vi "BIAS_Wrapper.vi"() -> ()   [LabVIEW 2012]
uses:
  <userlib>/bias2/subvis/ui/CameraParameters.ctl
  <userlib>/_OpenG.lib/array/array.llb/Search 1D Array (Boolean)__ogtk.vi
panel:
  in  "Labconfig file":path=path "C:/labconfig/ianspielman9339.ini"
  out "zlock port":u32=7339
  out "zlock server":string="atomchip-1.nist.gov"
  out "Current Camera":i32
  in  "Camera Select":i32(c297)
  out "Started":bool=TRUE
  out "VI refs":refnum<vi>[](array[refnum])
  in  "Location of BIAS vi":path=path "C:/Program Files (x86)/National Instruments/LabVIEW 2012/user.lib/BIAS2/BIAS_Client.vi"
  in  "offline":bool
  out "h5 file":path=path "C:/Experiments/rb_chip/connectiontable.h5"
  in  "cancel":bool
  in  "connect":bool
  in  "cameras":i32[](listbox)=[1]
  # "Global configuration options"
  # "Select camera(s) to connect to:"
  # "Loaded config information"
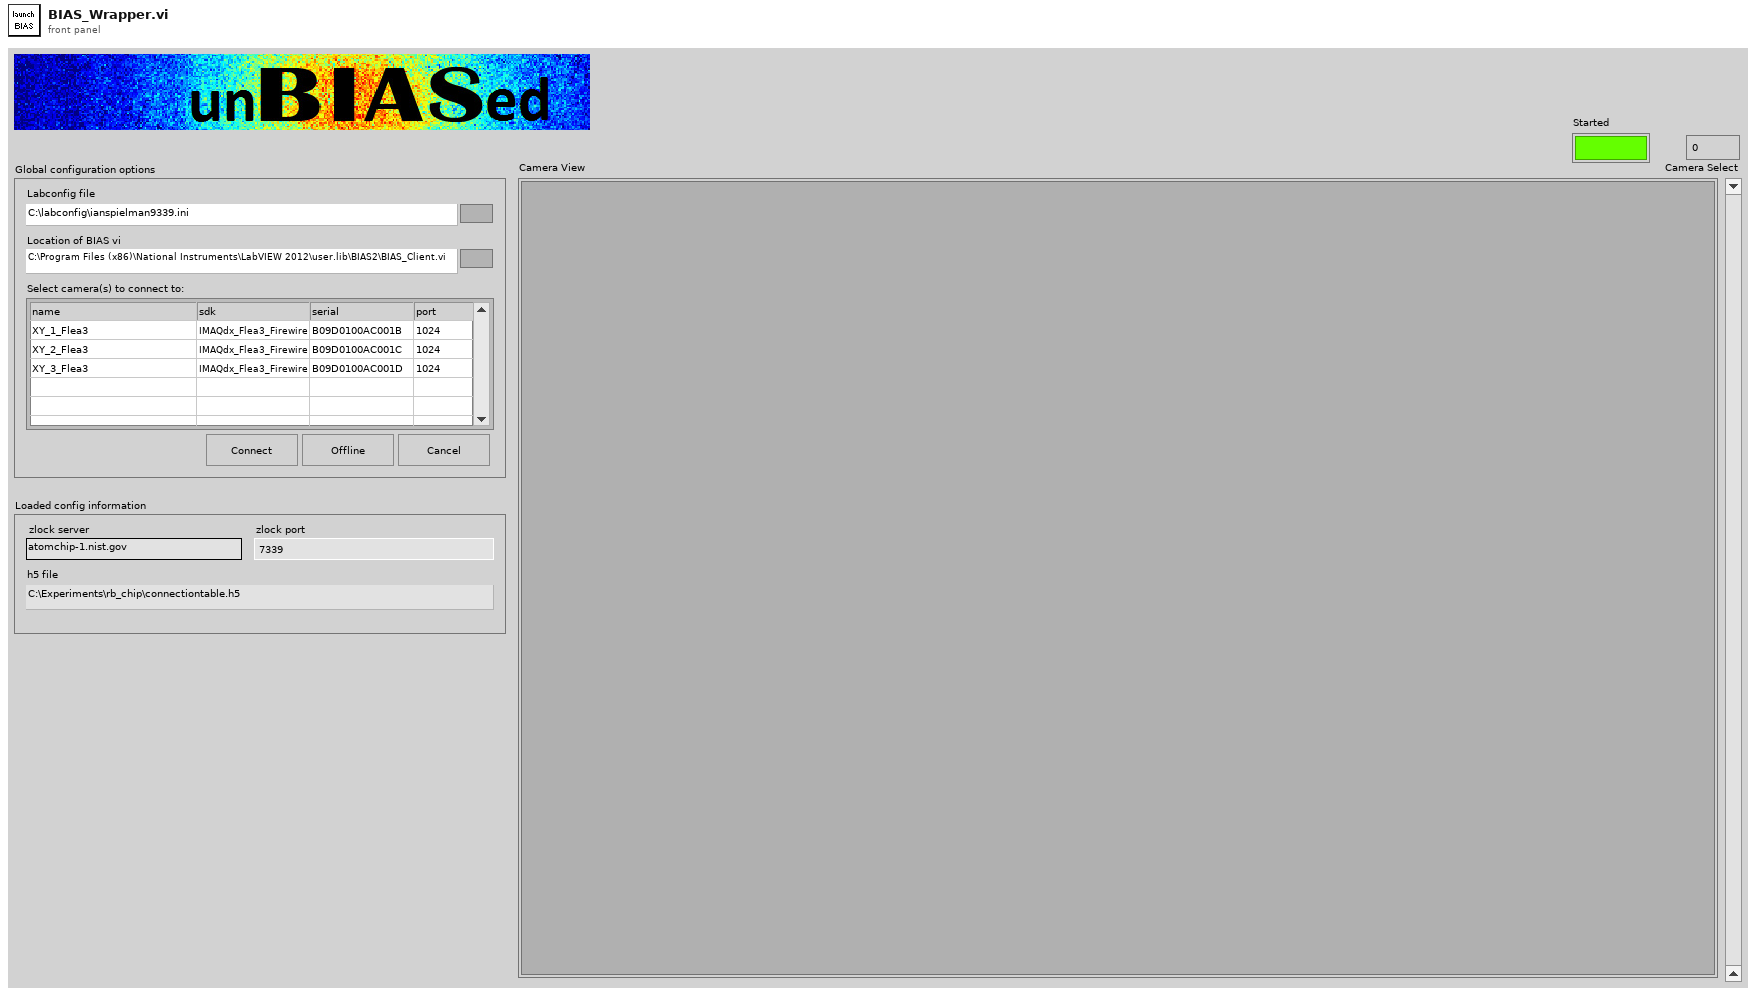
[diagram p1: front panel]
types:
  T1 = typedef "CameraParameters.ctl" = cluster{"name":string, "sdk":string, "serial":u64, "port":u16, "h5":path, "zlock server":string, "zlock port":u32}
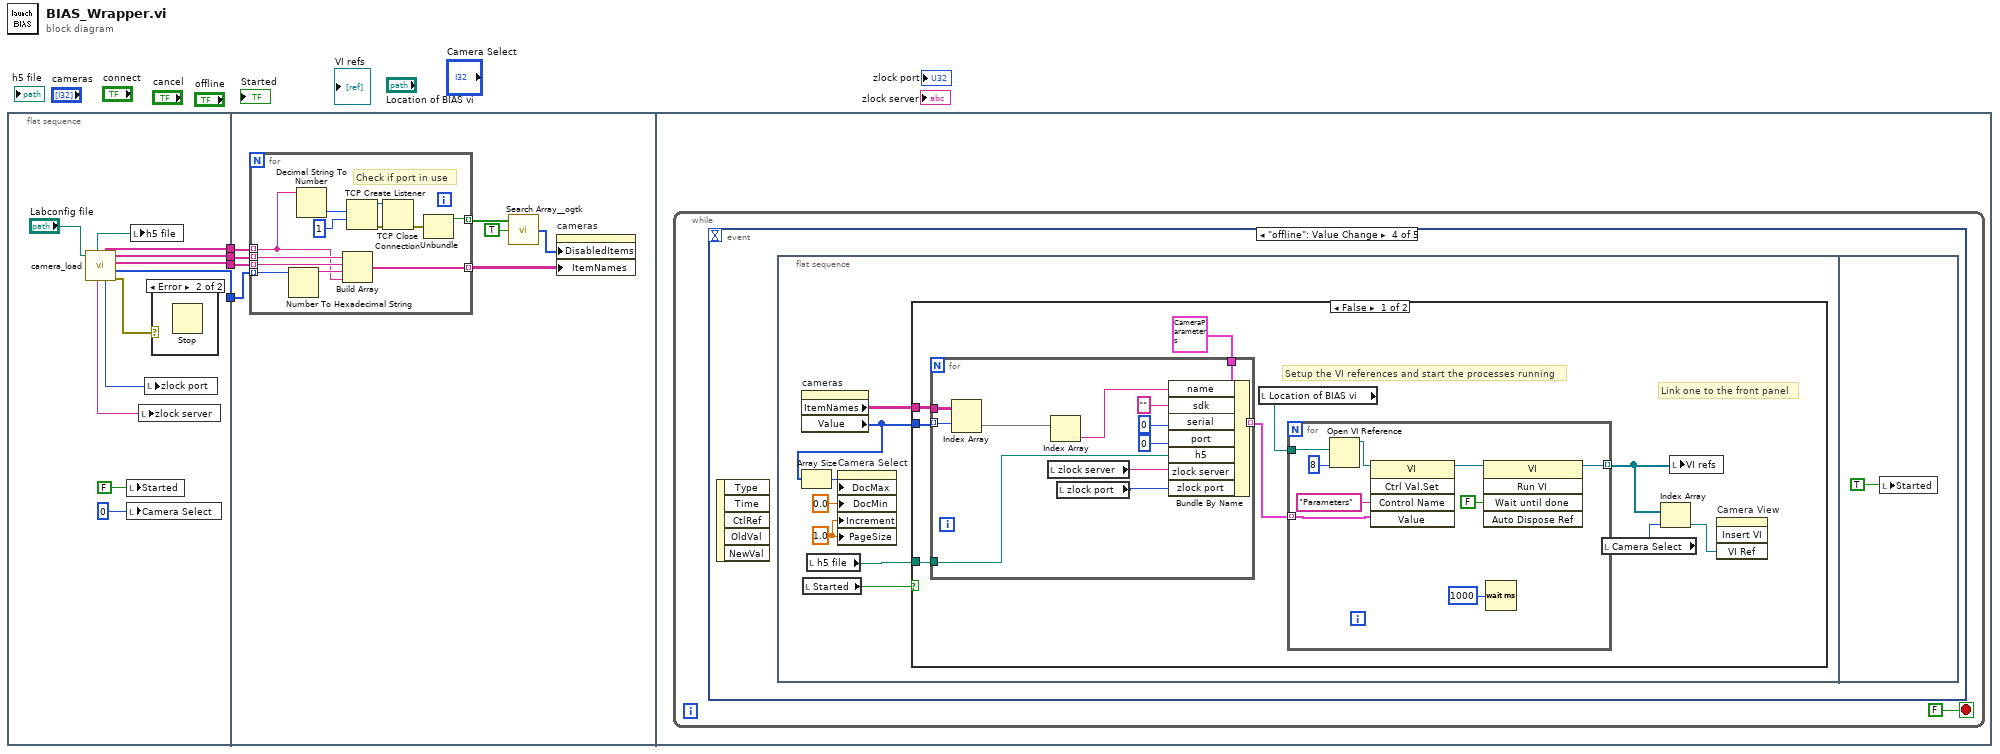
[diagram p0: block diagram]
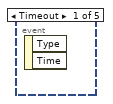
[diagram p3: hidden frame]
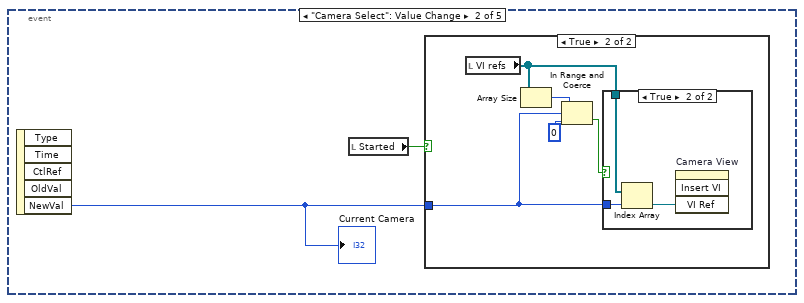
[diagram p4: hidden frame]
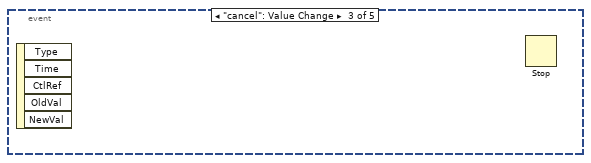
[diagram p7: hidden frame]
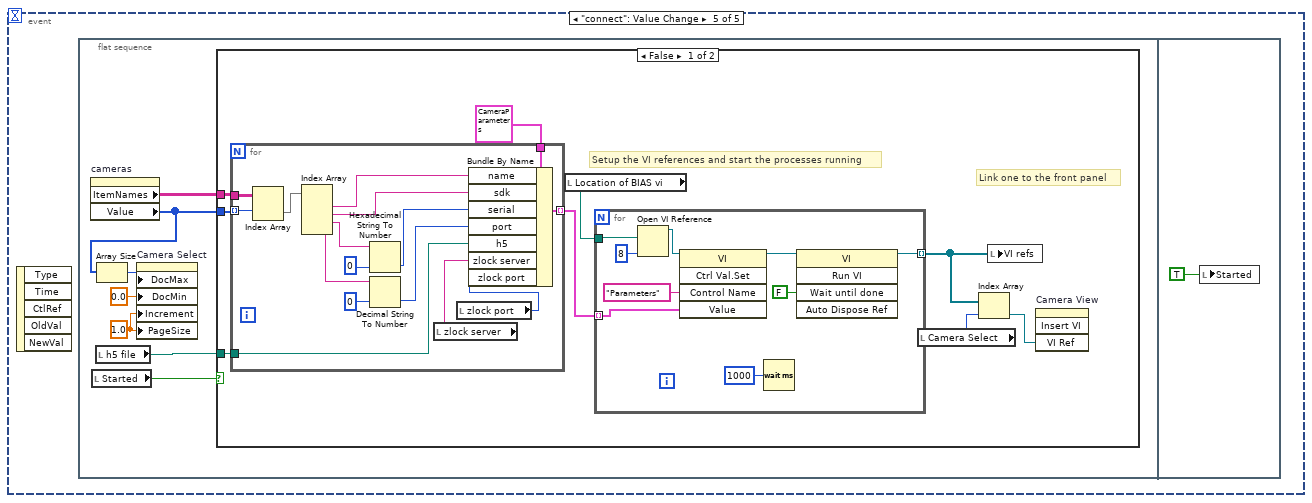
[diagram p9: hidden frame]
diagram:
  n1 = flat-sequence {
    tunnel: [w10] -> w4
    tunnel: [w11] -> w3
    tunnel: [w12] -> w2
    tunnel: [w13] -> w1
    tunnel: w4 -> [w23]
    tunnel: w3 -> [w22]
    tunnel: w2 -> [w21]
    tunnel: w1 -> [w20]
    frame #0 {
      n2 = call <userlib>:"camera_load.vi"("path"="Labconfig file") -> ("error out"=w8:errorcluster, "serials"=w10:u64[], "sdks"=w11:string[], "names"=w12:string[], "zlock port"=w5:u32, "ports"=w13:string[], "zlock server"=w6:string, "hdf"=w9:path)  [unwired: 3 in]
      n3 = local write "Started"(FALSE ("GO")) -> ()
      n4 = local write "Camera Select"(0 ("index")) -> ()
      n5 = local write "h5 file"(w9) -> ()
      n6 = local write "zlock server"(w6) -> ()
      n7 = local write "zlock port"(w5) -> ()
      n8 = case shown="Error" w8 {
        frame No Error {
        }
        frame Error {
          n9 = Stop() -> ()  [unwired: 1 in]
        }
      }
    }
    frame #1 {
      n10 = for {
        tunnel: w21 -> [w35] mode=indexing
        tunnel: w22 -> [w34] mode=indexing
        tunnel: w23 -> [w33] mode=indexing
        tunnel: [w31] -> w16 mode=indexing
        tunnel: w20 -> [w30] mode=indexing
        tunnel: [w24] -> w19 mode=indexing
        # "Check if port in use"
        n11 = Number To Hexadecimal String(2:w33) -> (0:w32:string)  [unwired: 1 in]
        n12 = Decimal String To Number(string=w30) -> (number=w29:i32)  [unwired: 2 in, 1 out]
        n13 = Build Array(w35, w34, w32, w30) -> (w31:string[])
        n14 = TCP Create Listener(9:1 ("timeout ms (25000)"), 10:w29) -> (0:w27:errorcluster, 3:w26:refnum<k5>)  [unwired: 3 in, 1 out]
        n15 = TCP Close Connection(connection ID=w26, error in (no error)=w27) -> (error out=w25:errorcluster)  [unwired: 1 in, 1 out]
        n16 = Unbundle(w25) -> ("status"=w24:bool)  [unwired: 2 out]
      }
      n17 = call-poly <userlib>:"Search Array__ogtk.vi"("Array"=w19, "Element Data"=TRUE) -> ("Indices of Elements"=w17:i32[])  [unwired: 7 in]
      n18 = property on="cameras" class="MCListbox (strict)"("DisabledItems"=w17, "ItemNames"=w16) -> ()  [unwired: 2 in, 2 out]
    }
    frame #2 {
      n19 = while {
        stop <- FALSE stop-if-true
        n20 = event shown="[3] \"offline\": Value Change" {
          selector: _ -> [_ _ _ _ _]
          dyn-events: _ -> [_ _ _ _ _]
          timeout: _ -> [_ _ _ _ _]
          event Timeout {
            n21 = event-data() -> ()  [unwired: 1 in, 2 out]
          }
          event "Camera Select": Value Change {
            n22 = event-data() -> ("NewVal"=w37:i32)  [unwired: 1 in, 4 out]
            "Current Camera" <- w37
            n23 = local read "Started"() -> (w38:bool)
            n24 = case shown="True" w38 {
              tunnel: w37 -> [_ w42]
              frame False {
              }
              frame True {
                n25 = local read "VI refs"() -> (w39:refnum<vi>[])
                n26 = Array Size(array=w39) -> (size(s)=w43:i32)
                n27 = In Range and Coerce(upper limit=w43, x=w42, lower limit=0) -> (In Range?=w40:bool)  [unwired: 1 out]
                n28 = case shown="True" w40 {
                  tunnel: w42 -> [_ w45]
                  tunnel: w39 -> [_ w44]
                  frame False {
                  }
                  frame True {
                    n29 = Index Array(array=w44, index=w45) -> (element=w46:refnum<vi>)
                    n30 = invoke on="Camera View" class="SubPnl" method="Insert VI"("VI Ref"=w46) -> ()  [unwired: 3 in, 4 out]
                  }
                }
              }
            }
          }
          event "cancel": Value Change {
            n31 = event-data() -> ()  [unwired: 1 in, 5 out]
            n32 = Stop() -> ()  [unwired: 1 in]
          }
          event "offline": Value Change {
            n33 = event-data() -> ()  [unwired: 1 in, 5 out]
            n34 = flat-sequence {
              frame #0 {
                w49 = 1.0 ("Increment")
                n35 = property on="cameras" class="MCListbox (strict)"() -> ("ItemNames"=w52:string[][], "Value"=w47:i32[])  [unwired: 2 in, 2 out]
                n36 = Array Size(array=w47) -> (size(s)=w48:i32)
                n37 = local read "Started"() -> (w53:bool)
                n38 = local read "h5 file"() -> (w51:path)
                n39 = property on="Camera Select" class="Scroll (strict)"("DocMax"=w48, "DocMin"=0.0 ("Doc Min"), "Increment"=w49, "PageSize"=w49) -> ()  [unwired: 2 in, 2 out]
                n40 = case shown="False" w53 {
                  tunnel: w52 -> [w61 _]
                  tunnel: w47 -> [w60 _]
                  tunnel: w51 -> [w62 _]
                  frame False {
                    # "Link one to the front panel"
                    # "Setup the VI references and start the processes running"
                    n41 = for {
                      tunnel: w61 -> [w83]
                      tunnel: w60 -> [w81] mode=indexing
                      tunnel: [w79] -> w55 mode=indexing
                      tunnel: T1 {"name"="", "sdk"="", "serial"=0, "port"=0, "h5"=path "", "zlock server"="atomchip-1.nist.gov", "zlock port"=0} ("Parameteres") -> [w78]
                      tunnel: w62 -> [w77]
                      n42 = Index Array(array=w83, index (row)=w81) -> (element=w82:string[])  [unwired: 1 in]
                      n43 = local read "zlock server"() -> (w72:string)
                      n44 = Index Array(array=w82) -> (element=w80:string)  [unwired: 1 in]
                      n45 = local read "zlock port"() -> (w73:u32)
                      n46 = Bundle By Name(cluster=w78, "name"=w80, "sdk"="", "serial"=u64 0, "port"=u16 0, "h5"=w77, "zlock server"=w72, "zlock port"=w73) -> (w79:T1)
                    }
                    n47 = local read "Location of BIAS vi"() -> (w57:path)
                    n48 = for {
                      tunnel: [w68] -> w56 mode=indexing
                      tunnel: w57 -> [w67]
                      tunnel: w55 -> [w64] mode=indexing
                      n49 = Open VI Reference(vi path=w67, options=8) -> (vi reference=w71:refnum<vi>)  [unwired: 4 in, 1 out]
                      n50 = invoke class="VI" method="Ctrl Val.Set"(reference=w71, "Control Name"="Parameters", "Value"=w64) -> (reference out=w66:refnum<vi>)  [unwired: 2 in, 4 out]
                      n51 = invoke class="VI" method="Run VI"(reference=w66, "Wait until done"=FALSE ("Wait Until Done")) -> (reference out=w68:refnum<vi>)  [unwired: 3 in, 4 out]
                      n52 = Wait (ms)(milliseconds to wait=u32 1000) -> ()  [unwired: 1 out]
                    }
                    n53 = local read "Camera Select"() -> (w59:i32)
                    n54 = Index Array(array=w56, index=w59) -> (element=w58:refnum<vi>)
                    n55 = local write "VI refs"(w56) -> ()
                    n56 = invoke on="Camera View" class="SubPnl" method="Insert VI"("VI Ref"=w58) -> ()  [unwired: 3 in, 4 out]
                  }
                  frame True {
                  }
                }
              }
              frame #1 {
                n57 = local write "Started"(TRUE ("GO")) -> ()
              }
            }
          }
          event "connect": Value Change {
            n58 = event-data() -> ()  [unwired: 1 in, 5 out]
            n59 = flat-sequence {
              frame #0 {
                w87 = 1.0 ("Increment")
                n60 = property on="cameras" class="MCListbox (strict)"() -> ("ItemNames"=w90:string[][], "Value"=w85:i32[])  [unwired: 2 in, 2 out]
                n61 = local read "Started"() -> (w91:bool)
                n62 = local read "h5 file"() -> (w89:path)
                n63 = Array Size(array=w85) -> (size(s)=w88:i32)
                n64 = property on="Camera Select" class="Scroll (strict)"("DocMax"=w88, "DocMin"=0.0 ("Doc Min"), "Increment"=w87, "PageSize"=w87) -> ()  [unwired: 2 in, 2 out]
                n65 = case shown="False" w91 {
                  tunnel: w90 -> [w99 _]
                  tunnel: w85 -> [w98 _]
                  tunnel: w89 -> [w100 _]
                  frame False {
                    # "Link one to the front panel"
                    # "Setup the VI references and start the processes running"
                    n66 = for {
                      tunnel: w99 -> [w125]
                      tunnel: w98 -> [w124] mode=indexing
                      tunnel: [w123] -> w93 mode=indexing
                      tunnel: T1 {"name"="XY_1_Flea3", "sdk"="IMAQdx_Flea3_Firewire", "serial"=49712223532875803, "port"=1024, "h5"=path "Y:/Experiments/rb_chip/connectiontable.h5", "zlock server"="atomchip-1.nist.gov", "zlock port"=0} ("Parameters") -> [w122]
                      tunnel: w100 -> [w121]
                      n67 = Index Array(array=w125, index (row)=w124) -> (element=w116:string[])  [unwired: 1 in]
                      n68 = Index Array(array=w116) -> (element #1=w115:string, element #2=w114:string, element #3=w118:string, element #4=w119:string)  [unwired: 4 in]
                      n69 = Hexadecimal String To Number(string=w118, default (0uL)=u64 0 ("default (0 U32)")) -> (number=w113:u64)  [unwired: 1 in, 1 out]
                      n70 = Decimal String To Number(string=w119, default (0L)=u16 0 ("default (0 I32)")) -> (number=w112:u16)  [unwired: 1 in, 1 out]
                      n71 = local read "zlock server"() -> (w111:string)
                      n72 = local read "zlock port"() -> (w110:u32)
                      n73 = Bundle By Name(cluster=w122, "name"=w115, "sdk"=w114, "serial"=w113, "port"=w112, "h5"=w121, "zlock server"=w111, "zlock port"=w110) -> (w123:T1)
                    }
                    n74 = local read "Location of BIAS vi"() -> (w96:path)
                    n75 = for {
                      tunnel: [w106] -> w97 mode=indexing
                      tunnel: w96 -> [w105]
                      tunnel: w93 -> [w102] mode=indexing
                      n76 = Open VI Reference(vi path=w105, options=8) -> (vi reference=w109:refnum<vi>)  [unwired: 4 in, 1 out]
                      n77 = invoke class="VI" method="Ctrl Val.Set"(reference=w109, "Control Name"="Parameters", "Value"=w102) -> (reference out=w104:refnum<vi>)  [unwired: 2 in, 4 out]
                      n78 = Wait (ms)(milliseconds to wait=u32 1000) -> ()  [unwired: 1 out]
                      n79 = invoke class="VI" method="Run VI"(reference=w104, "Wait until done"=FALSE ("Wait Until Done")) -> (reference out=w106:refnum<vi>)  [unwired: 3 in, 4 out]
                    }
                    n80 = local read "Camera Select"() -> (w94:i32)
                    n81 = Index Array(array=w97, index=w94) -> (element=w95:refnum<vi>)
                    n82 = local write "VI refs"(w97) -> ()
                    n83 = invoke on="Camera View" class="SubPnl" method="Insert VI"("VI Ref"=w95) -> ()  [unwired: 3 in, 4 out]
                  }
                  frame True {
                  }
                }
              }
              frame #1 {
                n84 = local write "Started"(TRUE ("GO")) -> ()
              }
            }
          }
        }
      }
    }
  }
